vi "DAQmx电压采集.vi"(7 "被测通道":tag="Dev1/ai0", 8 "error in":errorcluster caption="错误输入", 10 "设置":string[](array[string])=["160", "10", "0.02", "0.02", "0.1", "10", "J5", "J6"], 11 "参考通道":tag="Dev1/ai0") -> (0 "error out":errorcluster caption="错误输出", 1 "被测幅值":dbl[](array[numeric]), 2 "参考幅值":dbl format="%.2p", 4 "满足条件":bool)   [LabVIEW 2015]
uses:
  <vilib>/Utility/error.llb/DialogType.ctl
  <vilib>/DAQmx/read.llb/DAQmx Read (Analog 1D Wfm NChan NSamp).vi
  <vilib>/DAQmx/create/channels.llb/DAQmx Create Channel (AI-Voltage-Basic).vi
  <vilib>/DAQmx/create/channels.llb/DAQmx Create Channel (AI-Acceleration-Accelerometer).vi
  <vilib>/DAQmx/configure/timing.llb/DAQmx Timing (Sample Clock).vi
  <vilib>/DAQmx/miscellaneous.llb/DAQmx Fill In Error Info.vi
  <vilib>/measure/matone.llb/Extract Single Tone Information N Chan.vi
  <resource>/objmgr/daqmx.rc
  <vilib>/measure/NI_MAPro.lvlib
panel:
  out "实际采样率":dbl=1000.0 format="%0.2f"
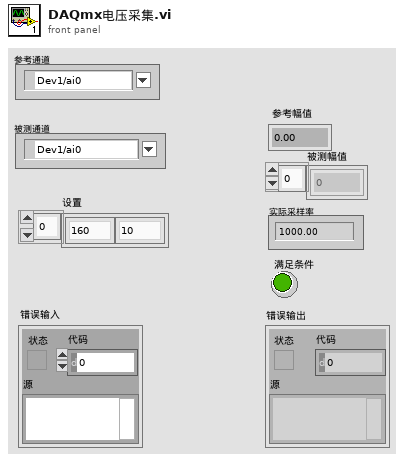
[diagram p1: front panel]
types:
  T1 = typedef "DialogType.ctl" = u16
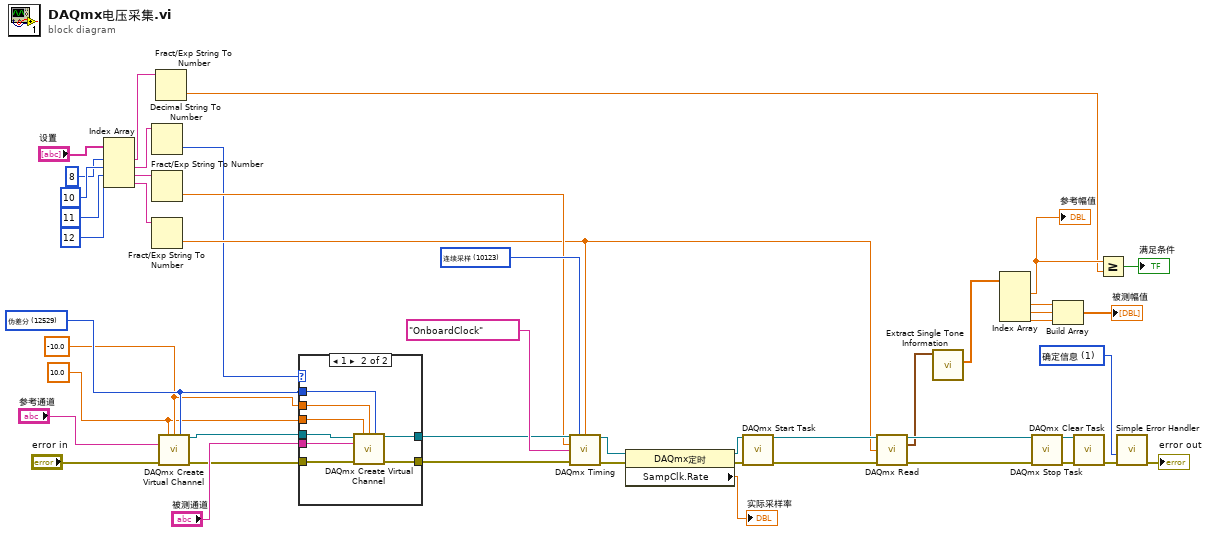
[diagram p0: block diagram]
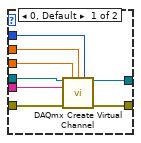
[diagram p2: hidden frame]
diagram:
  w36 = T1 1 items=["无对话框", "确定信息", "继续或停止信息", "确定信息＋警告", "继续/停止+警告"] ("type of dialog (OK msg:1)")
  w29 = 12529 items=["默认"=-1, "RSE"=10083, "NRSE"=10078, "差分"=10106, "伪差分"=12529] ("接线端配置")
  w27 = 10.0 ("最大电压")
  w28 = -10.0 ("最小电压")
  w47 = 10123 items=["有限采样"=10178, "连续采样"=10123, "硬件定时单点"=12522] ("sample mode")
  n1 = Index Array(array="设置", index #1=8 ("索引 (行)"), index #2=10 ("索引 (行)"), index #3=11 ("索引"), index #4=12 ("索引")) -> (element #1=w5:string, element #2=w13:string, element #3=w10:string, element #4=w7:string)
  n2 = Decimal String To Number(string=w13) -> (number=w17:i32)  [unwired: 2 in, 1 out]
  n3 = Fract/Exp String To Number(string=w10) -> (number=w19:dbl)  [unwired: 3 in, 1 out]
  n4 = Fract/Exp String To Number(string=w7) -> (number=w18:dbl)  [unwired: 3 in, 1 out]
  n5 = Fract/Exp String To Number(string=w5) -> (number=w15:dbl)  [unwired: 3 in, 1 out]
  n6 = call-poly <vilib>:"DAQmx Create Virtual Channel.vi"("maximum value"=w27, "minimum value"=w28, "input terminal configuration"=w29, "physical channels"="参考通道", "error in"="error in") -> ("task out"=w23:refnum<k21>, "error out"=w25:errorcluster)  [unwired: 9 in]
  n7 = case shown="1" w17 {
    tunnel: w29 -> [w55 w57]
    tunnel: w28 -> [w54 w58]
    tunnel: w27 -> [w53 w59]
    tunnel: w25 -> [w52 w62]
    tunnel: [w51 w60] -> w24
    tunnel: [w50 w61] -> w22
    tunnel: "被测通道" -> [w49 w63]
    tunnel: w23 -> [w48 w56]
    frame 0, Default {
      n8 = call-poly <vilib>:"DAQmx Create Virtual Channel.vi"("task in"=w48, "maximum value"=w53, "minimum value"=w54, "input terminal configuration"=w55, "physical channels"=w49, "error in"=w52) -> ("task out"=w50:refnum<k21>, "error out"=w51:errorcluster)  [unwired: 8 in]
    }
    frame 1 {
      n9 = call-poly <vilib>:"DAQmx Create Virtual Channel.vi"("task in"=w56, "maximum value"=w59, "minimum value"=w58, "input terminal configuration"=w57, "physical channels"=w63, "error in"=w62) -> ("task out"=w61:refnum<k21>, "error out"=w60:errorcluster)  [unwired: 8 in]
    }
  }
  n10 = call-poly <vilib>:"DAQmx Timing.vi"("task/channels in"=w22, "sample mode"=w47, "samples per channel"=w18, "rate"=w19, "source"=tag "OnboardClock" ("采样时钟源"), "error in"=w24) -> ("task out"=w38:refnum<k21>, "error out"=w41:errorcluster)  [unwired: 8 in]
  n11 = property class="DAQmx定时"(reference=w38, error in=w41) -> (reference out=w42:refnum<k21>, error out=w40:errorcluster, "SampClk.Rate"=→"实际采样率":dbl)
  n12 = call <vilib>:"DAQmx Start Task.vi"("task/channels in"=w42, "error in"=w40) -> ("task out"=w30:refnum<k21>, "error out"=w31:errorcluster)  [unwired: 12 in]
  n13 = call-poly <vilib>:"DAQmx Read.vi"("task/channels in"=w30, "number of samples per channel"=w18, "error in"=w31) -> ("task out"=w35:refnum<k21>, "data"=w21:waveform(dbl)[], "error out"=w32:errorcluster)  [unwired: 10 in]
  n14 = call-poly <vilib>:"Extract Single Tone Information.vi"("time signals in"=w21) -> ("detected amplitudes"=w20:dbl[])  [unwired: 5 in, 5 out]
  n15 = Index Array(array=w20) -> (element #1=w16:dbl, element #2=w4:dbl, element #3=w3:dbl, element #4=w2:dbl)  [unwired: 4 in]
  "参考幅值" <- w16
  n16 = call <vilib>:"DAQmx Stop Task.vi"("task/channels in"=w35, "error in"=w32) -> ("task out"=w34:refnum<k21>, "error out"=w33:errorcluster)  [unwired: 12 in]
  n17 = Build Array(w4, w3, w2) -> (→"被测幅值":dbl[])
  n18 = call <vilib>:"DAQmx Clear Task.vi"("task in"=w34, "error in"=w33) -> ("error out"=w37:errorcluster)  [unwired: 13 in]
  n19 = Greater Or Equal?(x=w16, y=w15) -> (x >= y?=→"满足条件":bool)
  n20 = call <vilib>:"Simple Error Handler.vi"("type of dialog (OK msg:1)"=w36, "error in (no error)"=w37) -> ("error out"=→"error out":errorcluster)  [unwired: 3 in, 4 out]
